vi "LockinRemoteControl.GetPrivateEvents.vi"(8 "error in (no error)":errorcluster, 11 "RemoteControl":refnum<class "LockinRemoteControl.lvclass">) -> (0 "error out":errorcluster, 2 "Private Events":T1, 3 "RemoteControl out":refnum<class "LockinRemoteControl.lvclass">)   [LabVIEW 2016, in "LockinRemoteControl.lvclass"]
doc: "---------------------------------------------------------------\nJKI State Machine Objects™\nhttp://jki.net/state-machine-objects/\nCopyright (C) 2005-2015, JKI <info@jki.net>\nALL RIGHTS RESERVEDJKI State Machine Objects (SMO) 1.0.0.4\nJKI - JKI\nCopyright (c) 2015, JKI"
uses:
  LockinRemoteControl.lvclass
  Typedefs/PrivateEvents--Cluster.ctl
  Typedefs/PrivateEvents--LockinRemoteControl.setAllowedRemoteAddress.ctl
  Typedefs/PrivateEvents--LockinRemoteControl.setAO.ctl
  Typedefs/PrivateEvents--LockinRemoteControl.setAI.ctl
  Typedefs/PrivateEvents--LockinRemoteControl.setResults.ctl
  Typedefs/PrivateEvents--LockinRemoteControl.setTrigger.ctl
  Typedefs/PrivateEvents--LockinRemoteControl.setAOconfig.ctl
  Typedefs/AO-cluster.ctl
  Typedefs/AO_Amp-array.ctl
  Typedefs/AO_DC-array.ctl
  Typedefs/AO_f-array.ctl
  Typedefs/AO_phi-array.ctl
  Typedefs/Function-array.ctl
  Typedefs/Function-enum.ctl
  Typedefs/PrivateEvents--LockinRemoteControl.setREFconfig.ctl
  Typedefs/REF-cluster.ctl
  Typedefs/REF_f-array.ctl
  Typedefs/REF_phi-array.ctl
  Typedefs/PrivateEvents--LockinRemoteControl.setReset.ctl
  Typedefs/PrivateEvents--LockinRemoteControl.setIVmode.ctl
  Typedefs/PrivateEvents--LockinRemoteControl.setREFfilterconfig.ctl
  Typedefs/REF filter-cluster.ctl
  Typedefs/PrivateEvents--LockinRemoteControl.setSamplingconfig.ctl
  LockinRemoteControl.lvclass/LockinRemoteControl.ctl
panel:
  # "For instructions on how to use the JKI State Machine Objects, examples and video tutorials, visit:\nhttp://jki.net/state-machine-objects/\n\nJKI State Machine Objects™\nhttp://jki.net/state-machine-objects/\nCopyright (C) 2005-2015, JKI <info@jki.net>\nALL RIGHTS RESERVED"
  # "1"
  # "2"
  # "3"
  # "4"
  # "5"
  # "6"
  # "7"
  # "8"
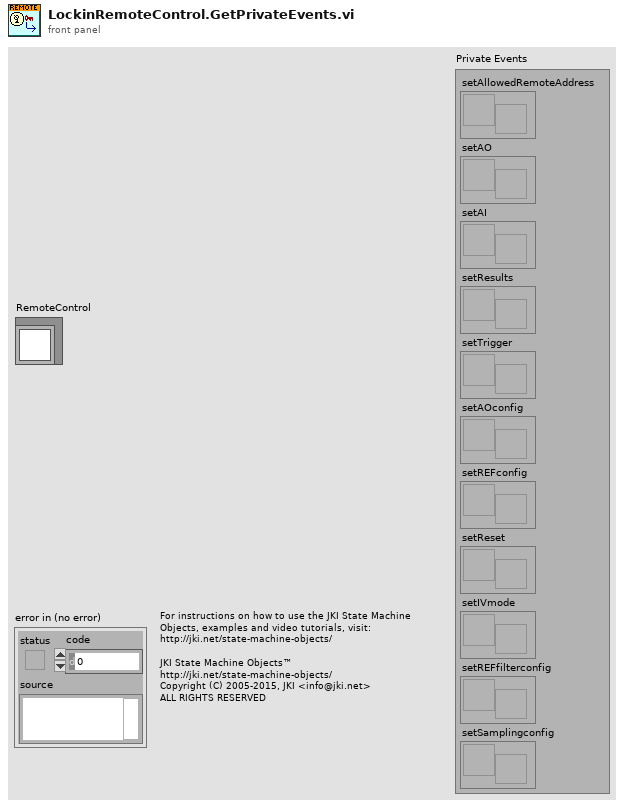
[diagram p1: front panel]
types:
  T1 = typedef "LockinRemoteControl.lvclass/PrivateEvents--Cluster.ctl" = cluster{"setAllowedRemoteAddress":refnum<user-event>, "setAO":refnum<user-event>, "setAI":refnum<user-event>, "setResults":refnum<user-event>, "setTrigger":refnum<user-event>, "setAOconfig":refnum<user-event>, "setREFconfig":refnum<user-event>, "setReset":refnum<user-event>, "setIVmode":refnum<user-event>, "setREFfilterconfig":refnum<user-event>, "setSamplingconfig":refnum<user-event>}
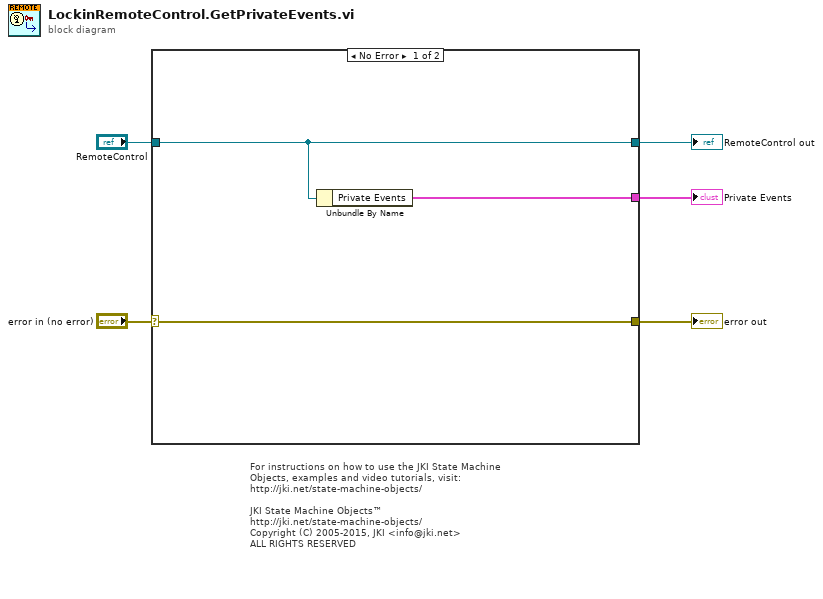
[diagram p0: block diagram]
diagram:
  # "For instructions on how to use the JKI State Machine Objects, examples and video tutorials, visit:\nhttp://jki.net/state-machine-objects/\n\nJKI State Machine Objects™\nhttp://jki.net/state-machine-objects/\nCopyright (C) 2005-2015, JKI <info@jki.net>\nALL RIGHTS RESERVED"
  n1 = case shown="No Error" "error in (no error)" {
    selector: "error in (no error)" -> [w7 w9]
    tunnel: "RemoteControl" -> [w6 w10]
    tunnel: [w7 w9] -> w4
    tunnel: [w6 w10] -> w3
    tunnel: [w8 _] -> w1
    frame No Error {
      n2 = Unbundle By Name(w6) -> ("Private Events"=w8:T1)
    }
    frame Error {
    }
  }
  "error out" <- w4
  "RemoteControl out" <- w3
  "Private Events" <- w1
